vi "EvaluateTriggerEnterCondition.vi"(7 "data group":string, 8 "error in":errorcluster, 10 "map":T1, 11 "operating states in":variant) -> (0 "error out":errorcluster, 1 "new operating state":i32, 3 "operating states out":variant, 4 "weight":i32)   [LabVIEW 2017, in "OpState.lvlib"]
uses:
  <vilib>/addons/InsightCM/Devices/Shared/Common/OpState/OpState.lvlib
  <vilib>/addons/PointValueMap/controls/PointMap.ctl
  <vilib>/addons/InsightCM/Devices/Shared/Common/OpState/controls/TriggerOperatingState.ctl
  <vilib>/addons/InsightCM/MessageBus/Base/controls/KeyValuePair.ctl
  <vilib>/addons/InsightCM/Devices/Shared/Common/Trigger/controls/TriggerCondition.ctl
  <vilib>/addons/InsightCM/MessageBus/Base/controls/Condition.ctl
  <vilib>/addons/InsightCM/Devices/Shared/Common/OpState/controls/ConditionType.ctl
  <vilib>/addons/InsightCM/Devices/Shared/Common/Trigger/Trigger.lvlib
  <vilib>/addons/InsightCM/Utilities/PropertyHelpers/PropertyHelpers.lvlib
  <vilib>/addons/PointValueMap/PointValueMap.lvlib
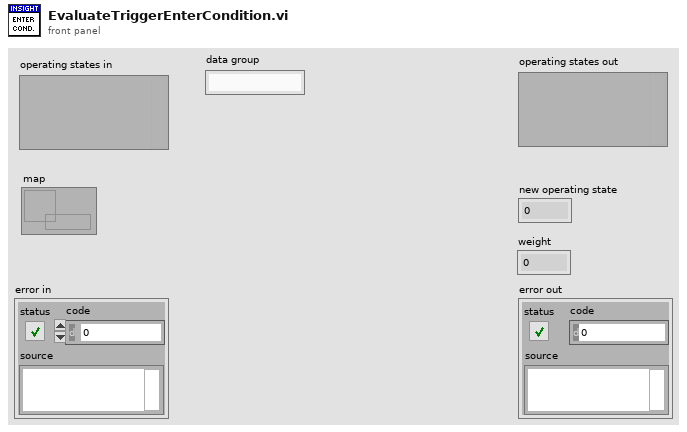
[diagram p1: front panel]
types:
  T1 = typedef "PointValueMap.lvlib/PointMap.ctl" = refnum<data-value>
  T2 = typedef "OpState.lvlib/TriggerOperatingState.ctl" = cluster{"Id":string, "Name":string, "Properties":T3[], "EnterExpression":string, "EnterConditions":T4[], "ExitExpression":string, "ExitConditions":T4[]}
  T3 = typedef "KeyValuePair.ctl" = cluster{"Key":string, "Value":string}
  T4 = typedef "Trigger.lvlib/TriggerCondition.ctl" = cluster{"Condition":T5, "LatchValue":string, "LatchTime":timestamp}
  T5 = typedef "Condition.ctl" = cluster{"Source":string, "Type":string, "Operator":string, "CompareTo":string, "DwellSeconds":dbl}
  T6 = typedef "OpState.lvlib/ConditionType.ctl" = enum16{"Enter", "Exit"}
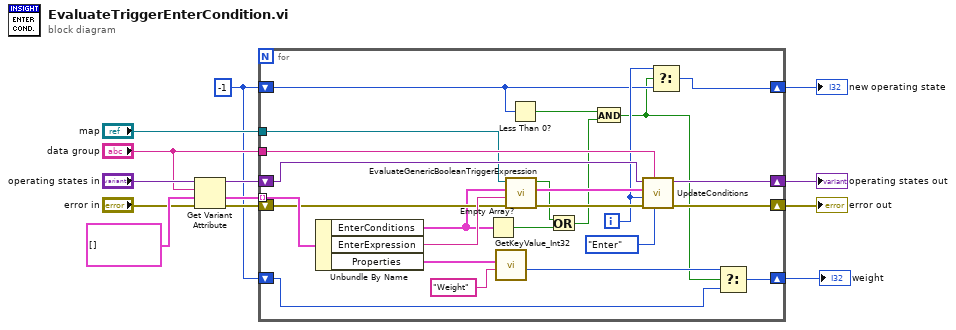
[diagram p0: block diagram]
diagram:
  w1 = -1
  n1 = Get Variant Attribute(Variant="operating states in", name="data group", default value (empty Variant)=T2[] [] ("OperatingStates"), error in="error in") -> (duplicate Variant=w8:variant, value=w4:T2[], error out=w9:errorcluster)  [unwired: 1 out]
  n2 = for {
    tunnel: "map" -> [w22]
    shift-right: [w20] -> w6
    shift-left: w9 -> [w32]
    shift-right: [w21] -> w7
    shift-left: w8 -> [w31]
    tunnel: "data group" -> [w36]
    tunnel: w4 -> [w34] mode=indexing
    shift-right: [w25] -> w3
    shift-left: w1 -> [w26]
    shift-right: [w16] -> w2
    shift-left: w1 -> [w14]
    i -> [w27]
    n3 = Unbundle By Name(w34) -> ("EnterConditions"=w30:T4[], "EnterExpression"=w33:string, "Properties"=w18:T3[])
    n4 = Empty Array?(array=w30) -> (empty?=w29:bool)
    n5 = call <vilib>:"GetKeyValue_Int32.vi"("key"="Weight", "key value pairs"=w18) -> ("value"=w17:i32)  [unwired: 7 in, 2 out]
    n6 = call <vilib>:"EvaluateGenericBooleanTriggerExpression.vi"("error in (no error)"=w32, "expression"=w33, "all conditions"=w30, "map"=w22) -> ("error out"=w37:errorcluster, "all conditions out"=w38:T4[], "trigger"=w24:bool)  [unwired: 4 in, 1 out]
    n7 = Less Than 0?(x=w26) -> (x < 0?=w28:bool)
    n8 = Or(x=w24, y=w29) -> (x .or. y?=w23:bool)
    n9 = And(x=w28, y=w23) -> (x .and. y?=w15:bool)
    n10 = call <vilib>:"UpdateConditions.vi"("ConditionType"=ConditionType."Enter", "data group"=w36, "error in (no error)"=w37, "OpState"=w27, "conditions"=w38, "operating states in"=w31) -> ("error out"=w20:errorcluster, "operating states out"=w21:variant)  [unwired: 4 in]
    n11 = Select(t=w27, s=w15, f=w26) -> (s? t:f=w25:i32)
    n12 = Select(t=w17, s=w15, f=w14) -> (s? t:f=w16:i32)
  }
  "error out" <- w6
  "operating states out" <- w7
  "new operating state" <- w3
  "weight" <- w2
